vi "S2C_PCIe7841_Proc_RefreshStatus.vi"(8 "Error In":errorcluster) -> (0 "Error Out":errorcluster)   [LabVIEW 2015]
uses:
  S2C_PCIe7841_Proc_Globals.vi
  <vilib>/Utility/error.llb/Error Cluster From Error Code.vi
  <vilib>/rvi/errors/niLvFpgaAdjustHostInterfaceError.vi
  <vilib>/rvi/interface/nirviReadWriteControl/nirviReadWriteControl.xnode
  NiFpgaLv.dll
  <vilib>/rvi/interface/Simulation/niFpgaSimulationCallBeginRW.vi
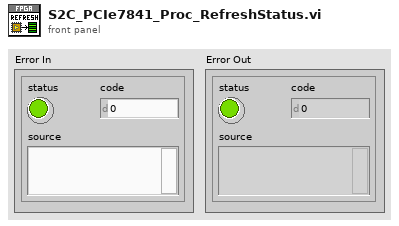
[diagram p1: front panel]
types:
  T1 = cluster{"Port 0":cluster{"P0B0":bool, "P0B1":bool, "P0B2":bool, "P0B3":bool, "P0B4":bool, "P0B5":bool, "P0B6":bool, "P0B7":bool}, "Port 1":cluster{"P1B0":bool, "P1B1":bool, "P1B2":bool, "P1B3":bool, "P1B4":bool, "P1B5":bool, "P1B6":bool, "P1B7":bool}, "Port 2":cluster{"P2B0":bool, "P2B1":bool, "P2B2":bool, "P2B3":bool, "P2B4":bool, "P2B5":bool, "P2B6":bool, "P2B7":bool}, "Port 3":cluster{"P3B0":bool, "P3B1":bool, "P3B2":bool, "P3B3":bool, "P3B4":bool, "P3B5":bool, "P3B6":bool, "P3B7":bool}, "Port 4":cluster{"P4B0":bool, "P4B1":bool, "P4B2":bool, "P4B3":bool, "P4B4":bool, "P4B5":bool, "P4B6":bool, "P4B7":bool}}
  T2 = cluster{"Port 0":cluster{"P0B0":bool, "P0B1":bool, "P0B2":bool, "P0B3":bool, "P0B4":bool, "P0B5":bool, "P0B6":bool, "P0B7":bool}, "Port 1":cluster{"P1B0":bool, "P1B1":bool, "P1B2":bool, "P1B3":bool, "P1B4":bool, "P1B5":bool, "P1B6":bool, "P1B7":bool}}
  T3 = cluster{"Boolean array[0]":bool, "Boolean array[1]":bool, "Boolean array[2]":bool, "Boolean array[3]":bool, "Boolean array[4]":bool, "Boolean array[5]":bool, "Boolean array[6]":bool, "Boolean array[7]":bool}
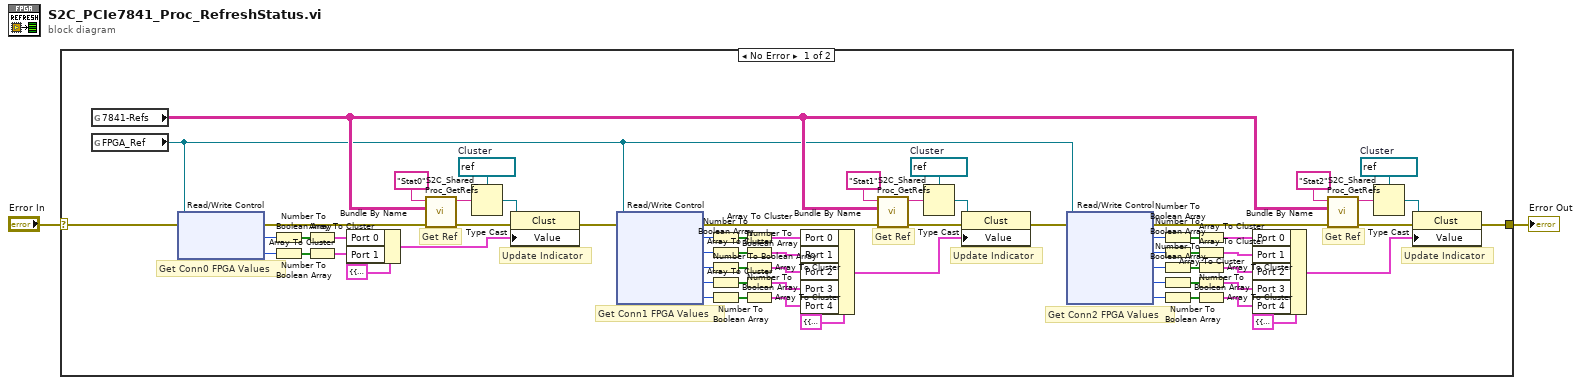
[diagram p0: block diagram]
diagram:
  n1 = case shown="No Error" "Error In" {
    selector: "Error In" -> [w45 w69]
    tunnel: [w50 w69] -> w1
    frame No Error {
      w56 = refnum<vi> refnum  # Cluster
      w57 = refnum<vi> refnum  # Cluster
      w68 = refnum<vi> refnum  # Cluster
      # "Update Indicator"
      # "Update Indicator"
      # "Update Indicator"
      # "Get Conn2 FPGA Values"
      # "Get Conn1 FPGA Values"
      # "Get Conn0 FPGA Values"
      # "Get Ref"
      # "Get Ref"
      # "Get Ref"
      n2 = global read "S2C_PCIe7841_Proc_Globals.vi" "7841-Refs"() -> (w51:string[][])
      n3 = global read "S2C_PCIe7841_Proc_Globals.vi" "FPGA_Ref"() -> (w4:refnum<k20>)
      n4 = xnode "Read/Write Control"("FPGA VI Reference In"=w4, "error in"=w45) -> ("error out"=w42:errorcluster, "Conn0/Port0"=w44:u8, "Conn0/Port1"=w43:u8)  [unwired: 1 out]
      n5 = Number To Boolean Array(number=w44) -> (Boolean array=w49:bool[])
      n6 = Number To Boolean Array(number=w43) -> (Boolean array=w47:bool[])
      n7 = Array To Cluster(array=w49) -> (cluster=w48:T3)
      n8 = Array To Cluster(array=w47) -> (cluster=w46:T3)
      n9 = Bundle By Name(cluster=T2 {"Port 0"={"P0B0"=FALSE, "P0B1"=FALSE, "P0B2"=FALSE, "P0B3"=FALSE, "P0B4"=FALSE, "P0B5"=FALSE, "P0B6"=FALSE, "P0B7"=FALSE}, "Port 1"={"P1B0"=FALSE, "P1B1"=FALSE, "P1B2"=FALSE, "P1B3"=FALSE, "P1B4"=FALSE, "P1B5"=FALSE, "P1B6"=FALSE, "P1B7"=FALSE}} ("Conn0"), "Port 0"=w48, "Port 1"=w46) -> (w63:T2)
      n10 = call "S2C_Shared_Proc_GetRefs.vi"("Error In"=w42, "Refs"=w51, "Label"="Stat0") -> ("Error Out"=w65:errorcluster, "Reference"=w67:string)  [unwired: 7 in]
      n11 = Type Cast(type=w68, x=w67) -> (*(type *) &x=w64:refnum<vi>)
      n12 = property class="Clust"(reference=w64, error in=w65, "Value"=w63) -> (error out=w31:errorcluster)  [unwired: 1 out]
      n13 = xnode "Read/Write Control"("FPGA VI Reference In"=w4, "error in"=w31) -> ("error out"=w30:errorcluster, "Conn1/Port0"=w39:u8, "Conn1/Port1"=w40:u8, "Conn1/Port2"=w34:u8, "Conn1/Port3"=w29:u8, "Conn1/Port4"=w32:u8)  [unwired: 1 out]
      n14 = Number To Boolean Array(number=w39) -> (Boolean array=w37:bool[])
      n15 = Number To Boolean Array(number=w40) -> (Boolean array=w38:bool[])
      n16 = Number To Boolean Array(number=w34) -> (Boolean array=w36:bool[])
      n17 = Number To Boolean Array(number=w29) -> (Boolean array=w35:bool[])
      n18 = Number To Boolean Array(number=w32) -> (Boolean array=w33:bool[])
      n19 = Array To Cluster(array=w37) -> (cluster=w27:T3)
      n20 = Array To Cluster(array=w38) -> (cluster=w23:T3)
      n21 = Array To Cluster(array=w36) -> (cluster=w24:T3)
      n22 = Array To Cluster(array=w35) -> (cluster=w25:T3)
      n23 = Array To Cluster(array=w33) -> (cluster=w26:T3)
      n24 = Bundle By Name(cluster=T1 {"Port 0"={"P0B0"=FALSE, "P0B1"=FALSE, "P0B2"=FALSE, "P0B3"=FALSE, "P0B4"=FALSE, "P0B5"=FALSE, "P0B6"=FALSE, "P0B7"=FALSE}, "Port 1"={"P1B0"=FALSE, "P1B1"=FALSE, "P1B2"=FALSE, "P1B3"=FALSE, "P1B4"=FALSE, "P1B5"=FALSE, "P1B6"=FALSE, "P1B7"=FALSE}, "Port 2"={"P2B0"=FALSE, "P2B1"=FALSE, "P2B2"=FALSE, "P2B3"=FALSE, "P2B4"=FALSE, "P2B5"=FALSE, "P2B6"=FALSE, "P2B7"=FALSE}, "Port 3"={"P3B0"=FALSE, "P3B1"=FALSE, "P3B2"=FALSE, "P3B3"=FALSE, "P3B4"=FALSE, "P3B5"=FALSE, "P3B6"=FALSE, "P3B7"=FALSE}, "Port 4"={"P4B0"=FALSE, "P4B1"=FALSE, "P4B2"=FALSE, "P4B3"=FALSE, "P4B4"=FALSE, "P4B5"=FALSE, "P4B6"=FALSE, "P4B7"=FALSE}} ("Conn1"), "Port 0"=w27, "Port 1"=w23, "Port 2"=w24, "Port 3"=w25, "Port 4"=w26) -> (w62:T1)
      n25 = call "S2C_Shared_Proc_GetRefs.vi"("Error In"=w30, "Refs"=w51, "Label"="Stat1") -> ("Error Out"=w60:errorcluster, "Reference"=w58:string)  [unwired: 7 in]
      n26 = Type Cast(type=w57, x=w58) -> (*(type *) &x=w61:refnum<vi>)
      n27 = property class="Clust"(reference=w61, error in=w60, "Value"=w62) -> (error out=w5:errorcluster)  [unwired: 1 out]
      n28 = xnode "Read/Write Control"("FPGA VI Reference In"=w4, "error in"=w5) -> ("error out"=w3:errorcluster, "Conn2/Port0"=w8:u8, "Conn2/Port1"=w7:u8, "Conn2/Port2"=w13:u8, "Conn2/Port3"=w16:u8, "Conn2/Port4"=w15:u8)  [unwired: 1 out]
      n29 = Number To Boolean Array(number=w8) -> (Boolean array=w10:bool[])
      n30 = Number To Boolean Array(number=w7) -> (Boolean array=w9:bool[])
      n31 = Number To Boolean Array(number=w13) -> (Boolean array=w11:bool[])
      n32 = Number To Boolean Array(number=w16) -> (Boolean array=w12:bool[])
      n33 = Number To Boolean Array(number=w15) -> (Boolean array=w14:bool[])
      n34 = Array To Cluster(array=w10) -> (cluster=w18:T3)
      n35 = Array To Cluster(array=w9) -> (cluster=w22:T3)
      n36 = Array To Cluster(array=w11) -> (cluster=w21:T3)
      n37 = Array To Cluster(array=w12) -> (cluster=w20:T3)
      n38 = Array To Cluster(array=w14) -> (cluster=w19:T3)
      n39 = Bundle By Name(cluster=T1 {"Port 0"={"P0B0"=FALSE, "P0B1"=FALSE, "P0B2"=FALSE, "P0B3"=FALSE, "P0B4"=FALSE, "P0B5"=FALSE, "P0B6"=FALSE, "P0B7"=FALSE}, "Port 1"={"P1B0"=FALSE, "P1B1"=FALSE, "P1B2"=FALSE, "P1B3"=FALSE, "P1B4"=FALSE, "P1B5"=FALSE, "P1B6"=FALSE, "P1B7"=FALSE}, "Port 2"={"P2B0"=FALSE, "P2B1"=FALSE, "P2B2"=FALSE, "P2B3"=FALSE, "P2B4"=FALSE, "P2B5"=FALSE, "P2B6"=FALSE, "P2B7"=FALSE}, "Port 3"={"P3B0"=FALSE, "P3B1"=FALSE, "P3B2"=FALSE, "P3B3"=FALSE, "P3B4"=FALSE, "P3B5"=FALSE, "P3B6"=FALSE, "P3B7"=FALSE}, "Port 4"={"P4B0"=FALSE, "P4B1"=FALSE, "P4B2"=FALSE, "P4B3"=FALSE, "P4B4"=FALSE, "P4B5"=FALSE, "P4B6"=FALSE, "P4B7"=FALSE}} ("Conn1"), "Port 0"=w18, "Port 1"=w22, "Port 2"=w21, "Port 3"=w20, "Port 4"=w19) -> (w6:T1)
      n40 = call "S2C_Shared_Proc_GetRefs.vi"("Error In"=w3, "Refs"=w51, "Label"="Stat2") -> ("Error Out"=w53:errorcluster, "Reference"=w55:string)  [unwired: 7 in]
      n41 = Type Cast(type=w56, x=w55) -> (*(type *) &x=w52:refnum<vi>)
      n42 = property class="Clust"(reference=w52, error in=w53, "Value"=w6) -> (error out=w50:errorcluster)  [unwired: 1 out]
    }
    frame Error {
    }
  }
  "Error Out" <- w1
